vi "get item names mclb.vi"(8 "error in (no error)":errorcluster, 10 "Control label":string, 11 "VI (Caller)":refnum<vi>) -> (0 "error out":errorcluster, 3 "Item names":string)   [LabVIEW 2020, in "ui-testing.lvlib"]
uses:
  ui-testing.lvlib
  <vilib>/addons/Tools/Unicode/UTF8 Tools.lvlib
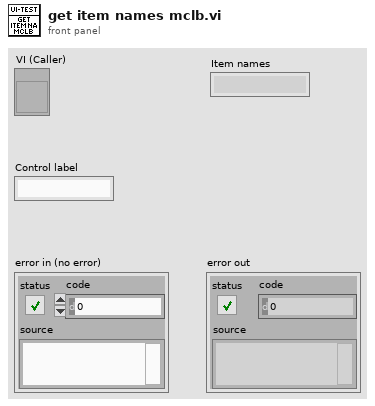
[diagram p1: front panel]
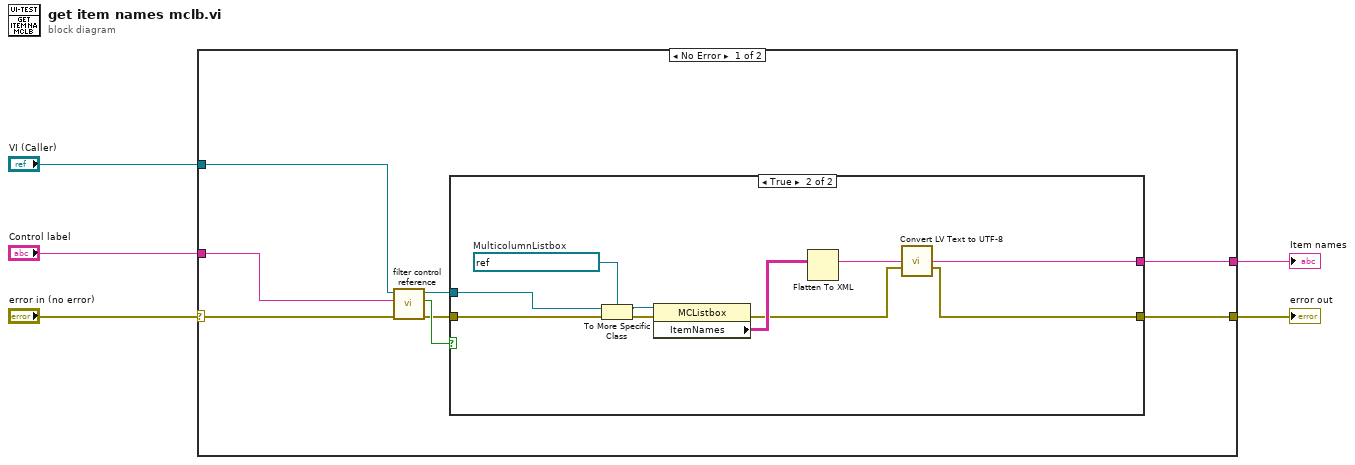
[diagram p0: block diagram]
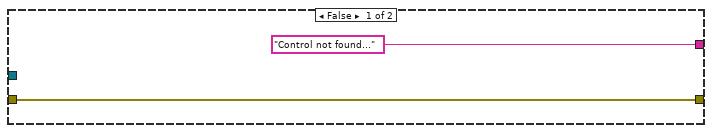
[diagram p2: hidden frame]
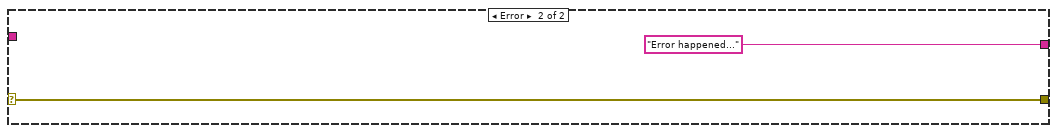
[diagram p3: hidden frame]
diagram:
  n1 = case shown="No Error" "error in (no error)" {
    selector: "error in (no error)" -> [w10 w27]
    tunnel: "Control label" -> [w9 _]
    tunnel: "VI (Caller)" -> [w8 _]
    tunnel: [w7 "Error happened..."] -> w2
    tunnel: [w6 w27] -> w1
    frame No Error {
      n2 = call "filter control reference.vi"("error in (no error)"=w10, "Control label"=w9, "VI (Caller)"=w8) -> ("error out"=w12:errorcluster, "Control found"=w13:bool, "Control ref"=w11:refnum<vi>)  [unwired: 6 in]
      n3 = case shown="True" w13 {
        tunnel: w12 -> [w15 w25]
        tunnel: w11 -> [_ w22]
        tunnel: ["Control not found..." w17] -> w7
        tunnel: [w15 w16] -> w6
        frame False {
        }
        frame True {
          w21 = refnum<vi> refnum  # MulticolumnListbox
          n4 = To More Specific Class(target class=w21, reference=w22, error in=w25) -> (specific class reference=w23:refnum<vi>, error out=w24:errorcluster)
          n5 = property class="MCListbox"(reference=w23, error in=w24) -> (error out=w18:errorcluster, "ItemNames"=w19:string[][])  [unwired: 1 out]
          n6 = Flatten To XML(6:w19) -> (2:w20:string)
          n7 = call <vilib>:"Convert LV Text to UTF-8.vi"("LV Text"=w20, "error in"=w18) -> ("UTF-8 Text"=w17:string, "error out"=w16:errorcluster)  [unwired: 12 in]
        }
      }
    }
    frame Error {
    }
  }
  "error out" <- w1
  "Item names" <- w2
